vi "search.vi"(5 "select-choice-software":T4, 7 "select-choice-location":string, 8 "View":string, 9 "Debug":bool, 11 "httpRequestID":u32) -> ()   [LabVIEW 2014]
uses:
  FRCts20_EspEngine.lvlib
  <vilib>/wsapi/NI_WebServices.lvlib
  <vilib>/wsapi/subVIs/Set Boolean ESP Variable.vi
  TypeDefs/FRCts20_EspEngine_SearchBrowser.ctl
  Web Methods/source/VI Source/Web Method Public Interface/FRCts20_WebMethods_ctl_teamIdentifier.ctl
  Web Methods/source/VI Source/FRCts20_WebMethods.lvlib
  Backend/source/VI Source/FRCts20_Backend_API/FRCts20_Backend_API_SW.ctl
  Web Methods/source/VI Source/Web Method Public Interface/FRCts20_WebMethods_ctl_singleEvent.ctl
  TypeDefs/FRCts20_EspEngine_Event.ctl
panel:
  in  "Event":T1={"Single Event"={"Team"=[{"Team Nickname"="Mark", "Team Number "=1, "UniqueId"=11}, {"Team Nickname"="Ryan", "Team Number "=2, "UniqueId"=22}, {"Team Nickname"="Whay", "Team Number "=5, "UniqueId"=55}, {"Team Nickname"="Jesse", "Team Number "=3, "UniqueId"=33}, {"Team Nickname"="Andrew", "Team Number "=4, "UniqueId"=44}], "Issue Count"=0, "Location"="", "Start Date "=timestamp(0 s since 1904-01-01)}, "EventOpenIssueCount"=0, "Requests"=[], "ClosedRequests"=[], "NotFoundStatus"=FALSE}
  out "error out":errorcluster
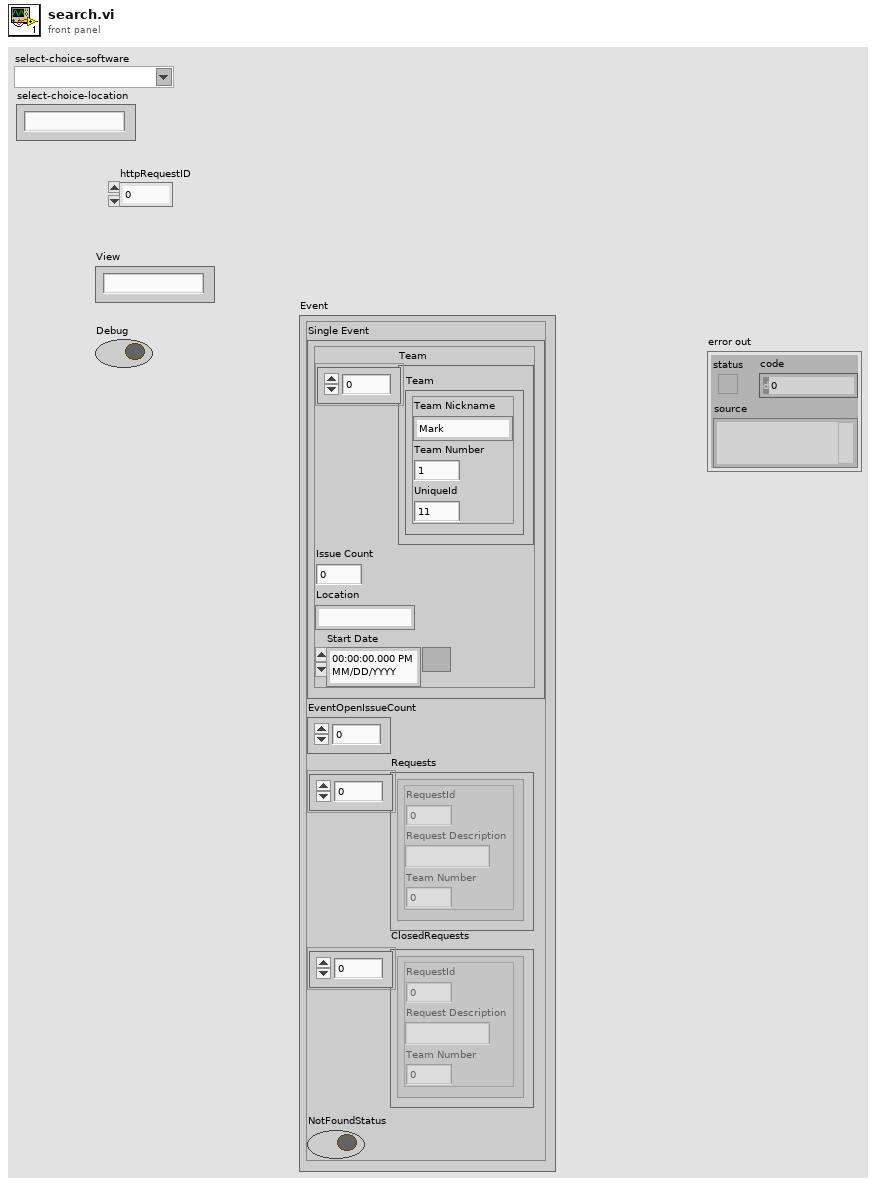
[diagram p1: front panel]
types:
  T1 = typedef "FRCts20_EspEngine.lvlib/FRCts20_EspEngine_Event.ctl" = cluster{"Single Event":T2, "EventOpenIssueCount":i16, "Requests":cluster{"RequestId":i32, "Request Description":string, "Team Number":i32}[], "ClosedRequests":cluster{"RequestId":i32, "Request Description":string, "Team Number":i32}[], "NotFoundStatus":bool}
  T2 = typedef "FRCts20_WebMethods.lvlib/FRCts20_WebMethods_ctl_singleEvent.ctl" = cluster{"Team":T3[], "Issue Count":i32, "Location":string, "Start Date ":timestamp}
  T3 = typedef "FRCts20_WebMethods.lvlib/FRCts20_WebMethods_ctl_teamIdentifier.ctl" = cluster{"Team Nickname":string, "Team Number ":u32, "UniqueId":u32}
  T4 = typedef "FRCts20_Backend_API.lvlib/FRCts20_Backend_API_SW.ctl" = string
  T5 = typedef "FRCts20_EspEngine.lvlib/FRCts20_EspEngine_SearchBrowser.ctl" = cluster{"Event":cluster{"Event Index":u32, "Event Name":string, "Start Time":timestamp, "End Time":timestamp, "OpenIssues":u8, "IsLive":bool}[], "select-choice-software":string, "select-choice-location":string}
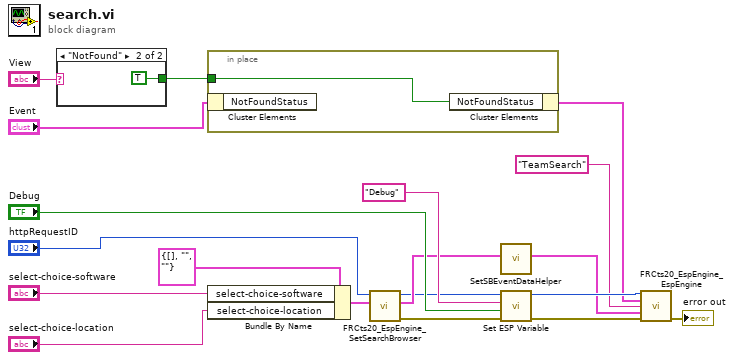
[diagram p0: block diagram]
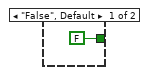
[diagram p2: hidden frame]
diagram:
  n1 = case shown="\"NotFound\"" "View" {
    tunnel: [FALSE TRUE] -> w8
    frame "False", Default {
    }
    frame "NotFound" {
    }
  }
  n2 = in-place {
    in-place-border: w8 -> [w22]
    n3 = in-place-cluster #1("Event") -> ()  [unwired: 1 out]
    n4 = in-place-cluster #1("NotFoundStatus"=w22) -> (w7:T1)
  }
  n5 = Bundle By Name(cluster=T5 {"Event"=[], "select-choice-software"="", "select-choice-location"=""} ("SearchBrowser"), "select-choice-software"="select-choice-software", "select-choice-location"="select-choice-location") -> (w3:T5)
  n6 = call "FRCts20_EspEngine_SetSearchBrowser.vi"("SearchBrowser"=w3, "httpRequestID"="httpRequestID") -> ("error out"=w11:errorcluster, "SearchBrowser"=w14:T5, "httpRequestID out"=w12:u32)  [unwired: 7 in]
  n7 = call "SetSBEventDataHelper.vi"("SearchBrowser"=w14) -> ("SearchBrowser"=w10:T5)  [unwired: 10 in]
  n8 = call-poly <vilib>:"Set ESP Variable.vi"("error in (no error)"=w11, "value"="Debug", "key"="Debug", "httpRequestID"=w12) -> ("error out"=w1:errorcluster, "httpRequestID out"=w17:u32)  [unwired: 6 in]
  n9 = call "FRCts20_EspEngine_EspEngine.vi"("httpRequestID"=w17, "Cluster"=w7, "Page"="TeamSearch", "SearchBrowser"=w10, "error in (no error)"=w1) -> ("error out"=→"error out":errorcluster)  [unwired: 9 in, 1 out]
